vi "24路数据解析例程.vi"() -> ()   [LabVIEW 2018]
panel:
  in  "16进制":bool
  in  "返回数据（字符串）":string
  out "LED IrCompare Result":u8[][](array[numeric])
  out "LED VfCompare Result":u8[][](array[numeric])
  out "LED IrResult":sgl[][](array[numeric]) format="%#_6f"
  out "LED VfResult":sgl[][](array[numeric]) format="%#_6f"
  out "Bls Result":sgl[][](array[numeric]) format="%#_6f"
  out "总判断":u8
  out "PS Compare Result":u8[][](array[numeric])
  out "Balance Compare Result":u8[][](array[numeric])
  out "Z Compare Result":u8[][](array[numeric])
  out "Rs Compare Result":u8[][](array[numeric])
  out "LxQ Compare Result":u8[][](array[numeric])
  out "DCR Compare Result":u8[][](array[numeric])
  out "C Compare Result":u8[][](array[numeric])
  out "Lk Compare Result":u8[][](array[numeric])
  out "Lx Compare Result":u8[][](array[numeric])
  out "Turns Compare Result":u8[][](array[numeric])
  out "Polarity Result1":string[][](array[string])
  out "Polarity Result":u8[][](array[numeric])
  out "Zx Result":sgl[][](array[numeric]) format="%#_6f"
  out "ACR Result":sgl[][](array[numeric]) format="%#_6f"
  out "LxQ Result":sgl[][](array[numeric]) format="%#_6f"
  out "DCR Result":sgl[][](array[numeric]) format="%#_6f"
  out "Cx Result":sgl[][](array[numeric]) format="%#_6f"
  out "Lk Result":sgl[][](array[numeric]) format="%#_6f"
  out "Lx Result":sgl[][](array[numeric]) format="%#_6f"
  out "Turns Result":sgl[][](array[numeric]) format="%#_6f"
  out "Primary Sets":string
  out "head":string
  in  "返回数据（16进制字符）":string
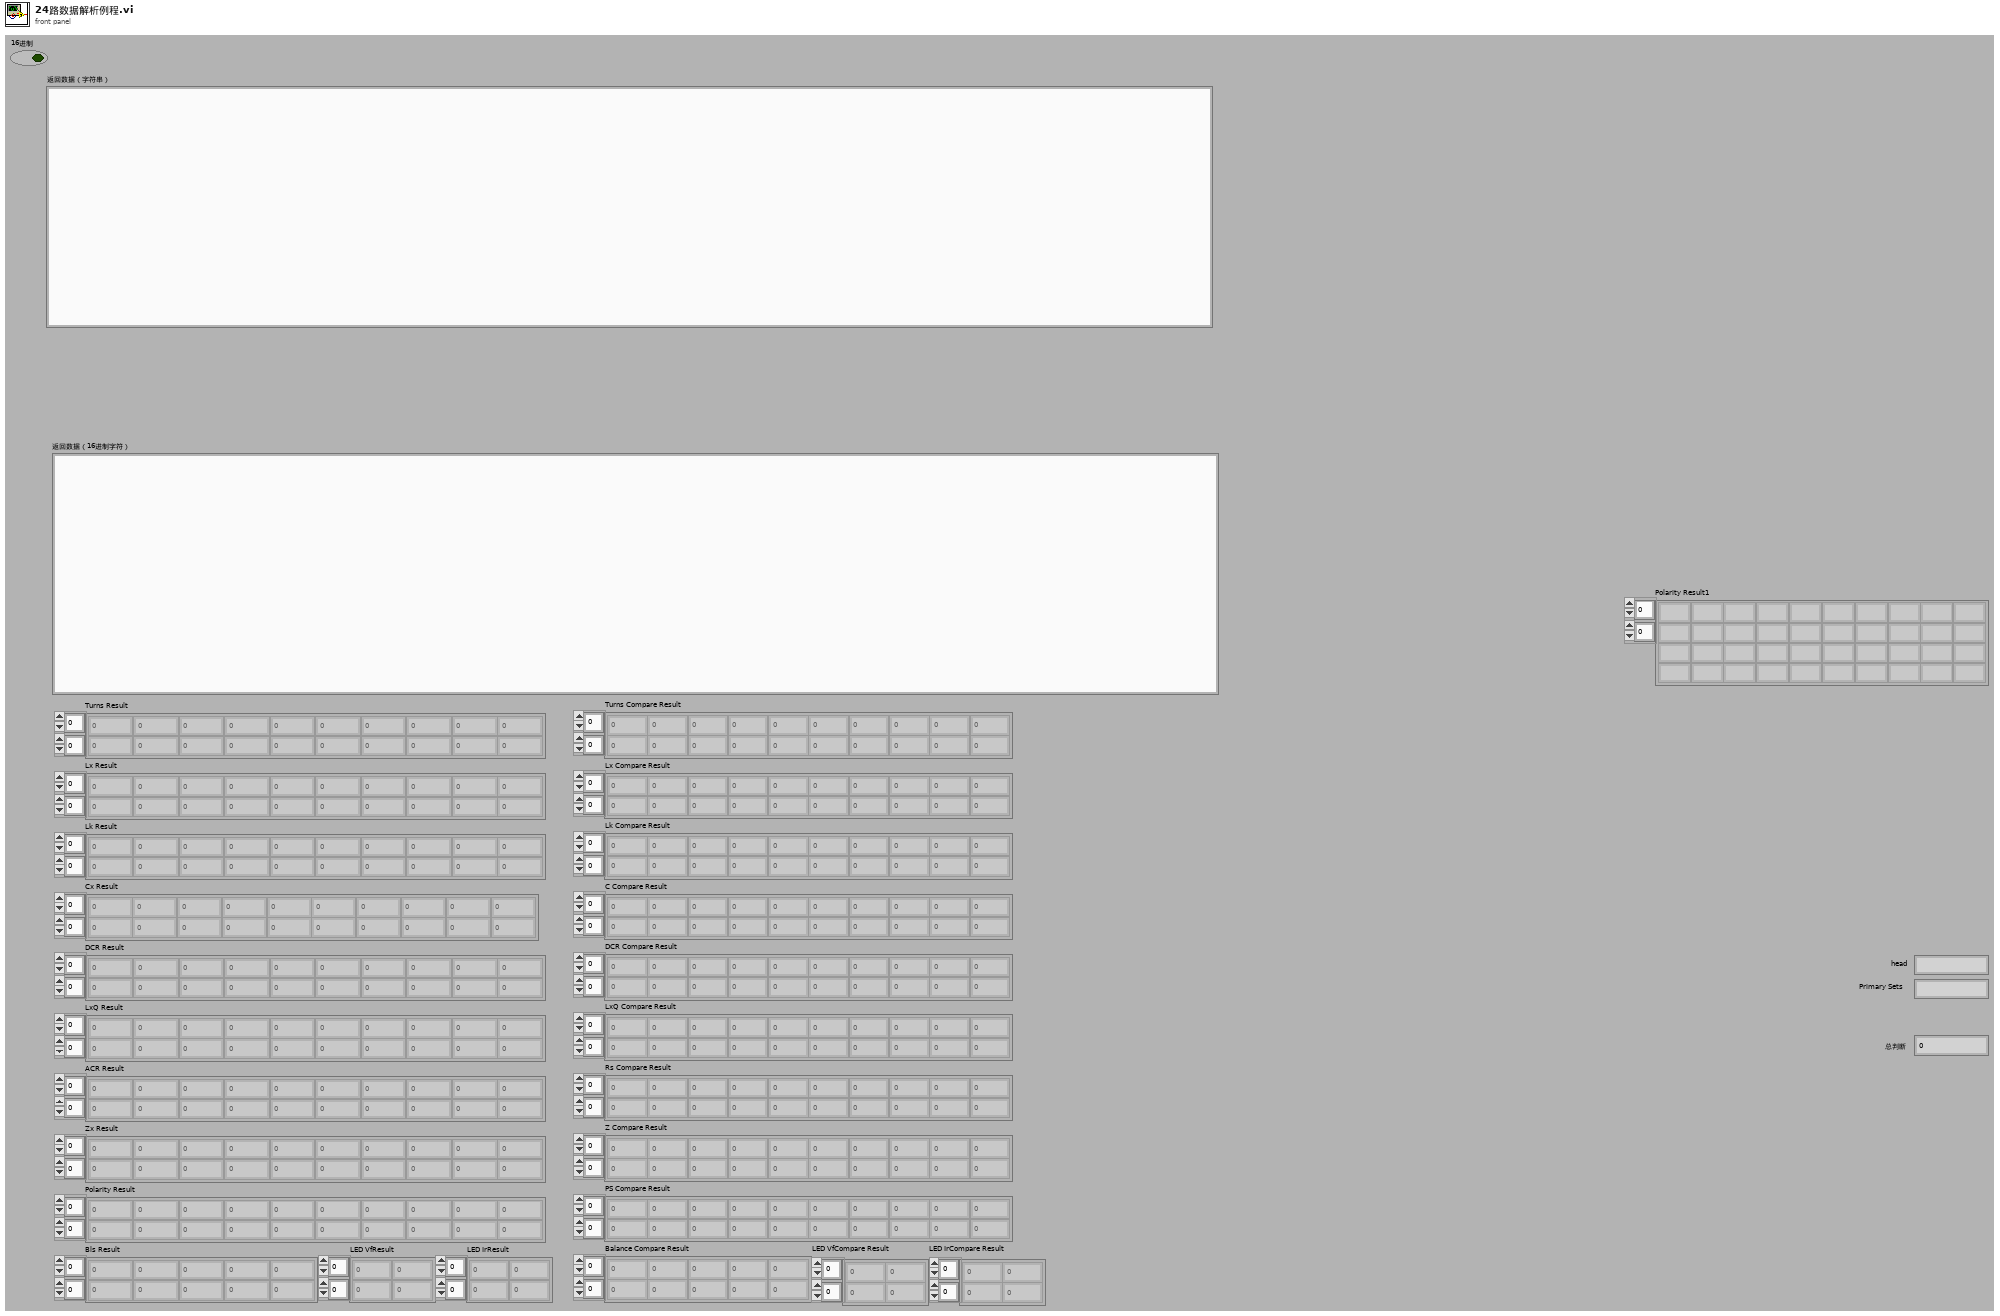
[diagram p1: front panel]
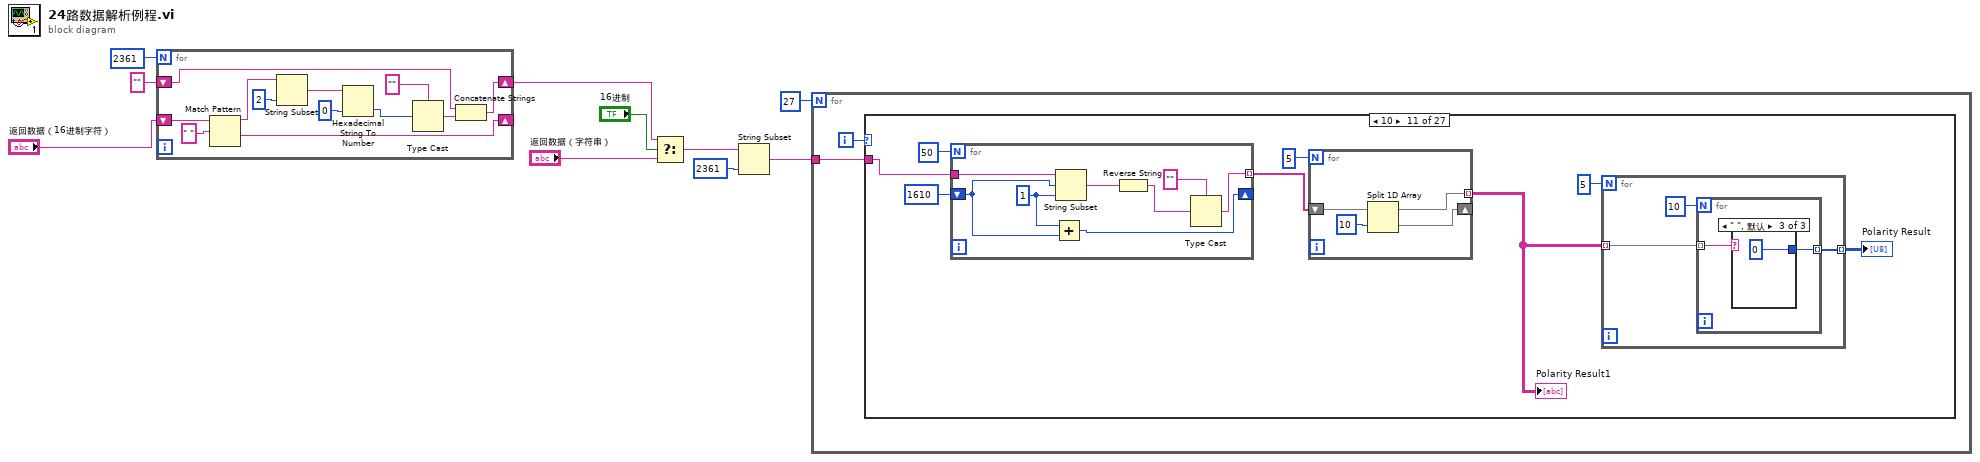
[diagram p0: block diagram]
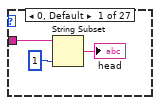
[diagram p2: hidden frame]
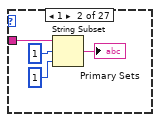
[diagram p3: hidden frame]
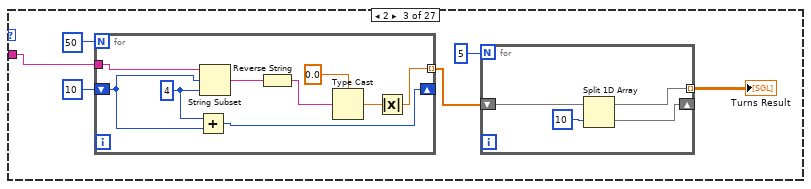
[diagram p4: hidden frame]
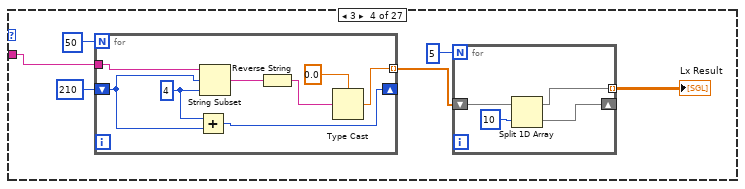
[diagram p5: hidden frame]
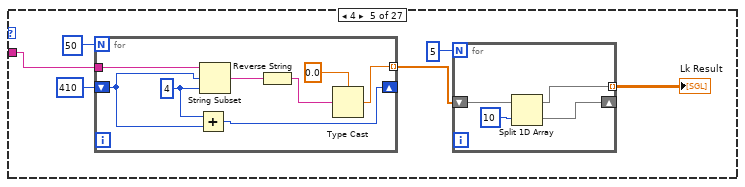
[diagram p6: hidden frame]
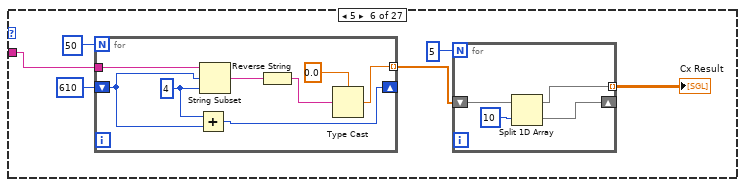
[diagram p7: hidden frame]
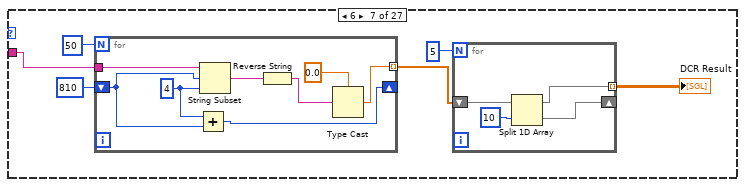
[diagram p8: hidden frame]
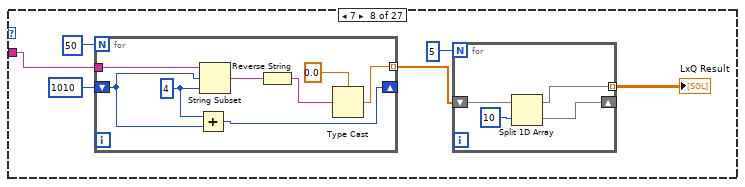
[diagram p9: hidden frame]
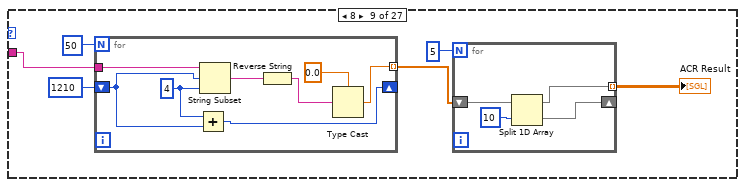
[diagram p10: hidden frame]
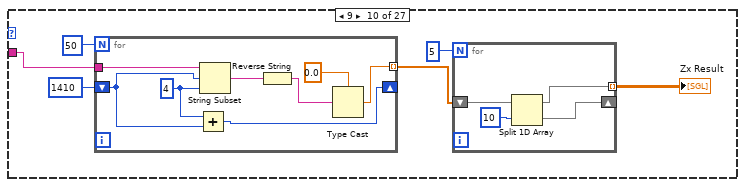
[diagram p11: hidden frame]
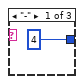
[diagram p12: hidden frame]
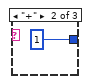
[diagram p13: hidden frame]
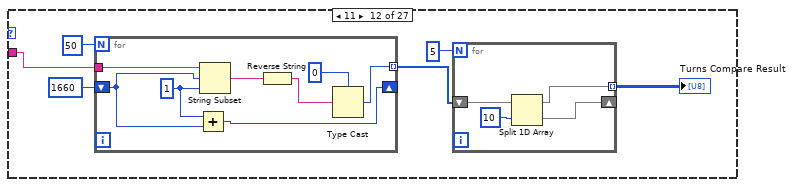
[diagram p14: hidden frame]
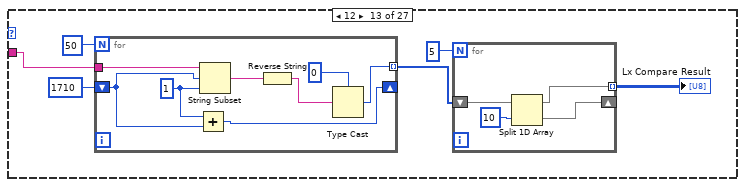
[diagram p15: hidden frame]
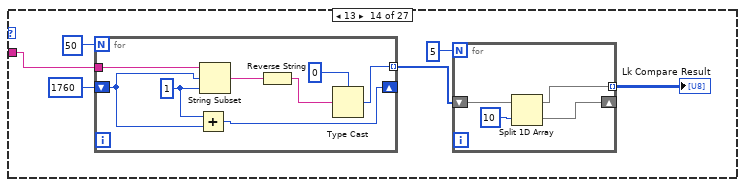
[diagram p16: hidden frame]
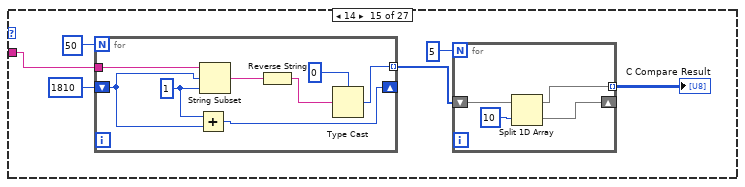
[diagram p17: hidden frame]
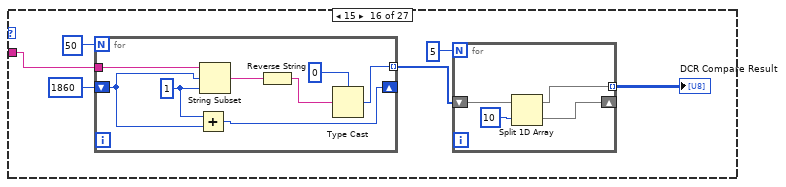
[diagram p18: hidden frame]
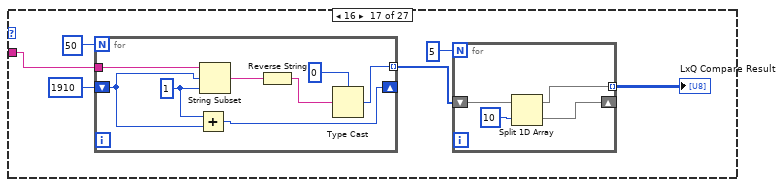
[diagram p19: hidden frame]
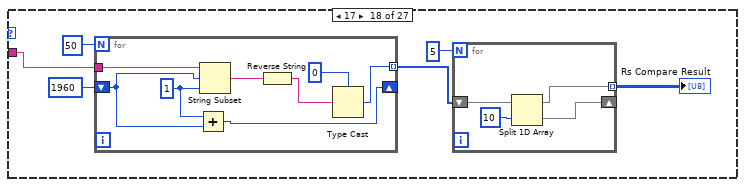
[diagram p20: hidden frame]
diagram:
  n1 = for {
    N: 2361 -> [_]
    shift-right: [w20] -> _
    shift-left: "返回数据（16进制字符）" -> [w22]
    shift-right: [w11] -> w4
    shift-left: "" -> [w13]
    n2 = Match Pattern(string=w22, regular expression=" " ("正则表达式")) -> (before substring=w16:string, after substring=w20:string)  [unwired: 1 in, 2 out]
    n3 = String Subset(string=w16, length (rest)=2 ("长度（剩余）")) -> (substring=w18:string)  [unwired: 1 in]
    n4 = Hexadecimal String To Number(string=w18, default (0uL)=u8 0 ("默认(0 U32)")) -> (number=w14:u8)  [unwired: 1 in, 1 out]
    n5 = Type Cast(type="", x=w14) -> (*(type *) &x=w12:string)
    n6 = Concatenate Strings(w13, w12) -> (w11:string)
  }
  n7 = Select(t=w4, s="16进制", f="返回数据（字符串）") -> (s? t:f=w1:string)
  n8 = String Subset(string=w1, length (rest)=2361 ("长度（剩余）")) -> (substring=w6:string)  [unwired: 1 in]
  n9 = for {
    N: 27 -> [_]
    tunnel: w6 -> [w23]
    i -> [w24]
    n10 = case shown="10" w24 {
      tunnel: w23 -> [w27 w31 w36 w55 w73 w91 w109 w127 w145 w163 w183 w209 w227 w245 w263 w281 w299 w317 w335 w353 w371 w388 w392 w410 w428 w446 w464]
      frame 0, Default {
        n11 = String Subset(string=w27, length (rest)=1 ("长度（剩余）")) -> (substring=→"head":string)  [unwired: 1 in]
      }
      frame 1 {
        n12 = String Subset ("截取字符串")(string=w31, offset (0)=1 ("长度（剩余）"), length (rest)=1 ("长度（剩余）")) -> (substring=→"Primary Sets":string)
      }
      frame 2 {
        n13 = for {
          N: 50 -> [_]
          shift-right: [w46] -> _
          shift-left: 10 ("长度（剩余）") -> [w42]
          tunnel: w36 -> [w41]
          tunnel: [w38] -> w34 mode=indexing
          w43 = 4 ("长度（剩余）")
          n14 = Add(x=w43, y=w42) -> (x+y=w46:i32)
          n15 = String Subset(string=w41, offset (0)=w42, length (rest)=w43) -> (substring=w40:string)
          n16 = Reverse String(1:w40) -> (0:w45:string)
          n17 = Type Cast(type=sgl 0.0 ("长度（剩余）"), x=w45) -> (*(type *) &x=w39:sgl)
          n18 = Absolute Value(x=w39) -> (abs(x)=w38:sgl)
        }
        n19 = for {
          N: 5 -> [_]
          shift-right: [w49] -> _
          shift-left: w34 -> [w47]
          tunnel: [w48] -> w32 mode=indexing
          n20 = Split 1D Array(array=w47, index=10 ("索引")) -> (first subarray=w48:sgl[], second subarray=w49:sgl[])
        }
        "Turns Result" <- w32
      }
      frame 3 {
        n21 = for {
          N: 50 -> [_]
          shift-right: [w64] -> _
          shift-left: 210 ("长度（剩余）") -> [w60]
          tunnel: w55 -> [w59]
          tunnel: [w57] -> w53 mode=indexing
          w61 = 4 ("长度（剩余）")
          n22 = Add(x=w61, y=w60) -> (x+y=w64:i32)
          n23 = String Subset(string=w59, offset (0)=w60, length (rest)=w61) -> (substring=w58:string)
          n24 = Reverse String(1:w58) -> (0:w63:string)
          n25 = Type Cast(type=sgl 0.0 ("长度（剩余）"), x=w63) -> (*(type *) &x=w57:sgl)
        }
        n26 = for {
          N: 5 -> [_]
          shift-right: [w67] -> _
          shift-left: w53 -> [w65]
          tunnel: [w66] -> w51 mode=indexing
          n27 = Split 1D Array(array=w65, index=10 ("索引")) -> (first subarray=w66:sgl[], second subarray=w67:sgl[])
        }
        "Lx Result" <- w51
      }
      frame 4 {
        n28 = for {
          N: 50 -> [_]
          shift-right: [w82] -> _
          shift-left: 410 ("长度（剩余）") -> [w78]
          tunnel: w73 -> [w77]
          tunnel: [w75] -> w71 mode=indexing
          w79 = 4 ("长度（剩余）")
          n29 = Add(x=w79, y=w78) -> (x+y=w82:i32)
          n30 = String Subset(string=w77, offset (0)=w78, length (rest)=w79) -> (substring=w76:string)
          n31 = Reverse String(1:w76) -> (0:w81:string)
          n32 = Type Cast(type=sgl 0.0 ("长度（剩余）"), x=w81) -> (*(type *) &x=w75:sgl)
        }
        n33 = for {
          N: 5 -> [_]
          shift-right: [w85] -> _
          shift-left: w71 -> [w83]
          tunnel: [w84] -> w69 mode=indexing
          n34 = Split 1D Array(array=w83, index=10 ("索引")) -> (first subarray=w84:sgl[], second subarray=w85:sgl[])
        }
        "Lk Result" <- w69
      }
      frame 5 {
        n35 = for {
          N: 50 -> [_]
          shift-right: [w100] -> _
          shift-left: 610 ("长度（剩余）") -> [w96]
          tunnel: w91 -> [w95]
          tunnel: [w93] -> w89 mode=indexing
          w97 = 4 ("长度（剩余）")
          n36 = Add(x=w97, y=w96) -> (x+y=w100:i32)
          n37 = String Subset(string=w95, offset (0)=w96, length (rest)=w97) -> (substring=w94:string)
          n38 = Reverse String(1:w94) -> (0:w99:string)
          n39 = Type Cast(type=sgl 0.0 ("长度（剩余）"), x=w99) -> (*(type *) &x=w93:sgl)
        }
        n40 = for {
          N: 5 -> [_]
          shift-right: [w103] -> _
          shift-left: w89 -> [w101]
          tunnel: [w102] -> w87 mode=indexing
          n41 = Split 1D Array(array=w101, index=10 ("索引")) -> (first subarray=w102:sgl[], second subarray=w103:sgl[])
        }
        "Cx Result" <- w87
      }
      frame 6 {
        n42 = for {
          N: 50 -> [_]
          shift-right: [w118] -> _
          shift-left: 810 ("长度（剩余）") -> [w114]
          tunnel: w109 -> [w113]
          tunnel: [w111] -> w107 mode=indexing
          w115 = 4 ("长度（剩余）")
          n43 = Add(x=w115, y=w114) -> (x+y=w118:i32)
          n44 = String Subset(string=w113, offset (0)=w114, length (rest)=w115) -> (substring=w112:string)
          n45 = Reverse String(1:w112) -> (0:w117:string)
          n46 = Type Cast(type=sgl 0.0 ("长度（剩余）"), x=w117) -> (*(type *) &x=w111:sgl)
        }
        n47 = for {
          N: 5 -> [_]
          shift-right: [w121] -> _
          shift-left: w107 -> [w119]
          tunnel: [w120] -> w105 mode=indexing
          n48 = Split 1D Array(array=w119, index=10 ("索引")) -> (first subarray=w120:sgl[], second subarray=w121:sgl[])
        }
        "DCR Result" <- w105
      }
      frame 7 {
        n49 = for {
          N: 50 -> [_]
          shift-right: [w136] -> _
          shift-left: 1010 ("长度（剩余）") -> [w132]
          tunnel: w127 -> [w131]
          tunnel: [w129] -> w125 mode=indexing
          w133 = 4 ("长度（剩余）")
          n50 = Add(x=w133, y=w132) -> (x+y=w136:i32)
          n51 = String Subset(string=w131, offset (0)=w132, length (rest)=w133) -> (substring=w130:string)
          n52 = Reverse String(1:w130) -> (0:w135:string)
          n53 = Type Cast(type=sgl 0.0 ("长度（剩余）"), x=w135) -> (*(type *) &x=w129:sgl)
        }
        n54 = for {
          N: 5 -> [_]
          shift-right: [w139] -> _
          shift-left: w125 -> [w137]
          tunnel: [w138] -> w123 mode=indexing
          n55 = Split 1D Array(array=w137, index=10 ("索引")) -> (first subarray=w138:sgl[], second subarray=w139:sgl[])
        }
        "LxQ Result" <- w123
      }
      frame 8 {
        n56 = for {
          N: 50 -> [_]
          shift-right: [w154] -> _
          shift-left: 1210 ("长度（剩余）") -> [w150]
          tunnel: w145 -> [w149]
          tunnel: [w147] -> w143 mode=indexing
          w151 = 4 ("长度（剩余）")
          n57 = Add(x=w151, y=w150) -> (x+y=w154:i32)
          n58 = String Subset(string=w149, offset (0)=w150, length (rest)=w151) -> (substring=w148:string)
          n59 = Reverse String(1:w148) -> (0:w153:string)
          n60 = Type Cast(type=sgl 0.0 ("长度（剩余）"), x=w153) -> (*(type *) &x=w147:sgl)
        }
        n61 = for {
          N: 5 -> [_]
          shift-right: [w157] -> _
          shift-left: w143 -> [w155]
          tunnel: [w156] -> w141 mode=indexing
          n62 = Split 1D Array(array=w155, index=10 ("索引")) -> (first subarray=w156:sgl[], second subarray=w157:sgl[])
        }
        "ACR Result" <- w141
      }
      frame 9 {
        n63 = for {
          N: 50 -> [_]
          shift-right: [w172] -> _
          shift-left: 1410 ("长度（剩余）") -> [w168]
          tunnel: w163 -> [w167]
          tunnel: [w165] -> w161 mode=indexing
          w169 = 4 ("长度（剩余）")
          n64 = Add(x=w169, y=w168) -> (x+y=w172:i32)
          n65 = String Subset(string=w167, offset (0)=w168, length (rest)=w169) -> (substring=w166:string)
          n66 = Reverse String(1:w166) -> (0:w171:string)
          n67 = Type Cast(type=sgl 0.0 ("长度（剩余）"), x=w171) -> (*(type *) &x=w165:sgl)
        }
        n68 = for {
          N: 5 -> [_]
          shift-right: [w175] -> _
          shift-left: w161 -> [w173]
          tunnel: [w174] -> w159 mode=indexing
          n69 = Split 1D Array(array=w173, index=10 ("索引")) -> (first subarray=w174:sgl[], second subarray=w175:sgl[])
        }
        "Zx Result" <- w159
      }
      frame 10 {
        n70 = for {
          N: 50 -> [_]
          shift-right: [w200] -> _
          shift-left: 1610 ("长度（剩余）") -> [w197]
          tunnel: w183 -> [w196]
          tunnel: [w194] -> w178 mode=indexing
          w198 = 1 ("长度（剩余）")
          n71 = Add(x=w198, y=w197) -> (x+y=w200:i32)
          n72 = String Subset(string=w196, offset (0)=w197, length (rest)=w198) -> (substring=w195:string)
          n73 = Reverse String(1:w195) -> (0:w199:string)
          n74 = Type Cast(type="", x=w199) -> (*(type *) &x=w194:string)
        }
        n75 = for {
          N: 5 -> [_]
          shift-right: [w203] -> _
          shift-left: w178 -> [w201]
          tunnel: [w202] -> w177 mode=indexing
          n76 = Split 1D Array(array=w201, index=10 ("索引")) -> (first subarray=w202:string[], second subarray=w203:string[])
        }
        "Polarity Result1" <- w177
        n77 = for {
          N: 5 -> [_]
          tunnel: w177 -> [w186] mode=indexing
          tunnel: [w185] -> w179 mode=indexing
          n78 = for {
            N: 10 -> [_]
            tunnel: w186 -> [w189] mode=indexing
            tunnel: [w188] -> w185 mode=indexing
            n79 = case shown="\" \", 默认" w189 {
              tunnel: [u8 4 u8 1 u8 0] -> w188
              frame "-" {
              }
              frame "+" {
              }
              frame " ", Default {
              }
            }
          }
        }
        "Polarity Result" <- w179
      }
      frame 11 {
        n80 = for {
          N: 50 -> [_]
          shift-right: [w218] -> _
          shift-left: 1660 ("长度（剩余）") -> [w214]
          tunnel: w209 -> [w213]
          tunnel: [w211] -> w207 mode=indexing
          w215 = 1 ("长度（剩余）")
          n81 = Add(x=w215, y=w214) -> (x+y=w218:i32)
          n82 = String Subset ("截取字符串")(string=w213, offset (0)=w214, length (rest)=w215) -> (substring=w212:string)
          n83 = Reverse String(1:w212) -> (0:w217:string)
          n84 = Type Cast(type=u8 0 ("长度（剩余）"), x=w217) -> (*(type *) &x=w211:u8)
        }
        n85 = for {
          N: 5 -> [_]
          shift-right: [w221] -> _
          shift-left: w207 -> [w219]
          tunnel: [w220] -> w205 mode=indexing
          n86 = Split 1D Array(array=w219, index=10 ("索引")) -> (first subarray=w220:u8[], second subarray=w221:u8[])
        }
        "Turns Compare Result" <- w205
      }
      frame 12 {
        n87 = for {
          N: 50 -> [_]
          shift-right: [w236] -> _
          shift-left: 1710 ("长度（剩余）") -> [w232]
          tunnel: w227 -> [w231]
          tunnel: [w229] -> w225 mode=indexing
          w233 = 1 ("长度（剩余）")
          n88 = Add(x=w233, y=w232) -> (x+y=w236:i32)
          n89 = String Subset(string=w231, offset (0)=w232, length (rest)=w233) -> (substring=w230:string)
          n90 = Reverse String(1:w230) -> (0:w235:string)
          n91 = Type Cast(type=u8 0 ("长度（剩余）"), x=w235) -> (*(type *) &x=w229:u8)
        }
        n92 = for {
          N: 5 -> [_]
          shift-right: [w239] -> _
          shift-left: w225 -> [w237]
          tunnel: [w238] -> w223 mode=indexing
          n93 = Split 1D Array(array=w237, index=10 ("索引")) -> (first subarray=w238:u8[], second subarray=w239:u8[])
        }
        "Lx Compare Result" <- w223
      }
      frame 13 {
        n94 = for {
          N: 50 -> [_]
          shift-right: [w254] -> _
          shift-left: 1760 ("长度（剩余）") -> [w250]
          tunnel: w245 -> [w249]
          tunnel: [w247] -> w243 mode=indexing
          w251 = 1 ("长度（剩余）")
          n95 = Add(x=w251, y=w250) -> (x+y=w254:i32)
          n96 = String Subset(string=w249, offset (0)=w250, length (rest)=w251) -> (substring=w248:string)
          n97 = Reverse String(1:w248) -> (0:w253:string)
          n98 = Type Cast(type=u8 0 ("长度（剩余）"), x=w253) -> (*(type *) &x=w247:u8)
        }
        n99 = for {
          N: 5 -> [_]
          shift-right: [w257] -> _
          shift-left: w243 -> [w255]
          tunnel: [w256] -> w241 mode=indexing
          n100 = Split 1D Array(array=w255, index=10 ("索引")) -> (first subarray=w256:u8[], second subarray=w257:u8[])
        }
        "Lk Compare Result" <- w241
      }
      frame 14 {
        n101 = for {
          N: 50 -> [_]
          shift-right: [w272] -> _
          shift-left: 1810 ("长度（剩余）") -> [w268]
          tunnel: w263 -> [w267]
          tunnel: [w265] -> w261 mode=indexing
          w269 = 1 ("长度（剩余）")
          n102 = Add(x=w269, y=w268) -> (x+y=w272:i32)
          n103 = String Subset(string=w267, offset (0)=w268, length (rest)=w269) -> (substring=w266:string)
          n104 = Reverse String(1:w266) -> (0:w271:string)
          n105 = Type Cast(type=u8 0 ("长度（剩余）"), x=w271) -> (*(type *) &x=w265:u8)
        }
        n106 = for {
          N: 5 -> [_]
          shift-right: [w275] -> _
          shift-left: w261 -> [w273]
          tunnel: [w274] -> w259 mode=indexing
          n107 = Split 1D Array(array=w273, index=10 ("索引")) -> (first subarray=w274:u8[], second subarray=w275:u8[])
        }
        "C Compare Result" <- w259
      }
      frame 15 {
        n108 = for {
          N: 50 -> [_]
          shift-right: [w290] -> _
          shift-left: 1860 ("长度（剩余）") -> [w286]
          tunnel: w281 -> [w285]
          tunnel: [w283] -> w279 mode=indexing
          w287 = 1 ("长度（剩余）")
          n109 = Add(x=w287, y=w286) -> (x+y=w290:i32)
          n110 = String Subset(string=w285, offset (0)=w286, length (rest)=w287) -> (substring=w284:string)
          n111 = Reverse String(1:w284) -> (0:w289:string)
          n112 = Type Cast(type=u8 0 ("长度（剩余）"), x=w289) -> (*(type *) &x=w283:u8)
        }
        n113 = for {
          N: 5 -> [_]
          shift-right: [w293] -> _
          shift-left: w279 -> [w291]
          tunnel: [w292] -> w277 mode=indexing
          n114 = Split 1D Array(array=w291, index=10 ("索引")) -> (first subarray=w292:u8[], second subarray=w293:u8[])
        }
        "DCR Compare Result" <- w277
      }
      frame 16 {
        n115 = for {
          N: 50 -> [_]
          shift-right: [w308] -> _
          shift-left: 1910 ("长度（剩余）") -> [w304]
          tunnel: w299 -> [w303]
          tunnel: [w301] -> w297 mode=indexing
          w305 = 1 ("长度（剩余）")
          n116 = Add(x=w305, y=w304) -> (x+y=w308:i32)
          n117 = String Subset(string=w303, offset (0)=w304, length (rest)=w305) -> (substring=w302:string)
          n118 = Reverse String(1:w302) -> (0:w307:string)
          n119 = Type Cast(type=u8 0 ("长度（剩余）"), x=w307) -> (*(type *) &x=w301:u8)
        }
        n120 = for {
          N: 5 -> [_]
          shift-right: [w311] -> _
          shift-left: w297 -> [w309]
          tunnel: [w310] -> w295 mode=indexing
          n121 = Split 1D Array(array=w309, index=10 ("索引")) -> (first subarray=w310:u8[], second subarray=w311:u8[])
        }
        "LxQ Compare Result" <- w295
      }
      frame 17 {
        n122 = for {
          N: 50 -> [_]
          shift-right: [w326] -> _
          shift-left: 1960 ("长度（剩余）") -> [w320]
          tunnel: w317 -> [w321]
          tunnel: [w322] -> w315 mode=indexing
          w319 = 1 ("长度（剩余）")
          n123 = Add(x=w319, y=w320) -> (x+y=w326:i32)
          n124 = String Subset(string=w321, offset (0)=w320, length (rest)=w319) -> (substring=w323:string)
          n125 = Reverse String(1:w323) -> (0:w325:string)
          n126 = Type Cast(type=u8 0 ("长度（剩余）"), x=w325) -> (*(type *) &x=w322:u8)
        }
        n127 = for {
          N: 5 -> [_]
          shift-right: [w329] -> _
          shift-left: w315 -> [w327]
          tunnel: [w328] -> w313 mode=indexing
          n128 = Split 1D Array(array=w327, index=10 ("索引")) -> (first subarray=w328:u8[], second subarray=w329:u8[])
        }
        "Rs Compare Result" <- w313
      }
      frame 18 {
        n129 = for {
          N: 50 -> [_]
          shift-right: [w344] -> _
          shift-left: 2010 ("长度（剩余）") -> [w338]
          tunnel: w335 -> [w339]
          tunnel: [w340] -> w333 mode=indexing
          w337 = 1 ("长度（剩余）")
          n130 = Add(x=w337, y=w338) -> (x+y=w344:i32)
          n131 = String Subset(string=w339, offset (0)=w338, length (rest)=w337) -> (substring=w341:string)
          n132 = Reverse String(1:w341) -> (0:w343:string)
          n133 = Type Cast(type=u8 0 ("长度（剩余）"), x=w343) -> (*(type *) &x=w340:u8)
        }
        n134 = for {
          N: 5 -> [_]
          shift-right: [w347] -> _
          shift-left: w333 -> [w345]
          tunnel: [w346] -> w331 mode=indexing
          n135 = Split 1D Array(array=w345, index=10 ("索引")) -> (first subarray=w346:u8[], second subarray=w347:u8[])
        }
        "Z Compare Result" <- w331
      }
      frame 19 {
        n136 = for {
          N: 50 -> [_]
          shift-right: [w362] -> _
          shift-left: 2060 ("长度（剩余）") -> [w357]
          tunnel: w353 -> [w358]
          tunnel: [w359] -> w351 mode=indexing
          w356 = 1 ("长度（剩余）")
          n137 = Add(x=w356, y=w357) -> (x+y=w362:i32)
          n138 = String Subset(string=w358, offset (0)=w357, length (rest)=w356) -> (substring=w360:string)
          n139 = Reverse String(1:w360) -> (0:w361:string)
          n140 = Type Cast(type=u8 0 ("长度（剩余）"), x=w361) -> (*(type *) &x=w359:u8)
        }
        n141 = for {
          N: 5 -> [_]
          shift-right: [w365] -> _
          shift-left: w351 -> [w363]
          tunnel: [w364] -> w349 mode=indexing
          n142 = Split 1D Array(array=w363, index=10 ("索引")) -> (first subarray=w364:u8[], second subarray=w365:u8[])
        }
        "Balance Compare Result" <- w349
      }
      frame 20 {
        n143 = for {
          N: 50 -> [_]
          shift-right: [w380] -> _
          shift-left: 2110 ("长度（剩余）") -> [w375]
          tunnel: w371 -> [w376]
          tunnel: [w377] -> w369 mode=indexing
          w374 = 1 ("长度（剩余）")
          n144 = Add(x=w374, y=w375) -> (x+y=w380:i32)
          n145 = String Subset(string=w376, offset (0)=w375, length (rest)=w374) -> (substring=w378:string)
          n146 = Reverse String(1:w378) -> (0:w379:string)
          n147 = Type Cast(type=u8 0 ("长度（剩余）"), x=w379) -> (*(type *) &x=w377:u8)
        }
        n148 = for {
          N: 5 -> [_]
          shift-right: [w383] -> _
          shift-left: w369 -> [w381]
          tunnel: [w382] -> w367 mode=indexing
          n149 = Split 1D Array(array=w381, index=10 ("索引")) -> (first subarray=w382:u8[], second subarray=w383:u8[])
        }
        "PS Compare Result" <- w367
      }
      frame 21 {
        n150 = String Subset(string=w388, offset (0)=2160 ("长度（剩余）"), length (rest)=1 ("长度（剩余）")) -> (substring=w391:string)
        n151 = Reverse String(1:w391) -> (0:w389:string)
        n152 = Type Cast(type=u8 0 ("长度（剩余）"), x=w389) -> (*(type *) &x=→"总判断":u8)
      }
      frame 22 {
        n153 = for {
          N: 25 -> [_]
          shift-right: [w405] -> _
          shift-left: 2161 ("长度（剩余）") -> [w401]
          tunnel: w392 -> [w400]
          tunnel: [w398] -> w395 mode=indexing
          w402 = 4 ("长度（剩余）")
          n154 = Add(x=w402, y=w401) -> (x+y=w405:i32)
          n155 = String Subset(string=w400, offset (0)=w401, length (rest)=w402) -> (substring=w399:string)
          n156 = Reverse String(1:w399) -> (0:w404:string)
          n157 = Type Cast(type=sgl 0.0 ("长度（剩余）"), x=w404) -> (*(type *) &x=w398:sgl)
        }
        n158 = for {
          N: 5 -> [_]
          shift-right: [w408] -> _
          shift-left: w395 -> [w406]
          tunnel: [w407] -> w393 mode=indexing
          n159 = Split 1D Array(array=w406, index=5 ("索引")) -> (first subarray=w407:sgl[], second subarray=w408:sgl[])
        }
        "Bls Result" <- w393
      }
      frame 23 {
        n160 = for {
          N: 10 -> [_]
          shift-right: [w423] -> _
          shift-left: 2261 ("长度（剩余）") -> [w419]
          tunnel: w410 -> [w418]
          tunnel: [w416] -> w412 mode=indexing
          w420 = 4 ("长度（剩余）")
          n161 = Add(x=w420, y=w419) -> (x+y=w423:i32)
          n162 = String Subset(string=w418, offset (0)=w419, length (rest)=w420) -> (substring=w417:string)
          n163 = Reverse String(1:w417) -> (0:w422:string)
          n164 = Type Cast(type=sgl 0.0 ("长度（剩余）"), x=w422) -> (*(type *) &x=w416:sgl)
        }
        n165 = for {
          N: 5 -> [_]
          shift-right: [w426] -> _
          shift-left: w412 -> [w424]
          tunnel: [w425] -> w415 mode=indexing
          n166 = Split 1D Array(array=w424, index=2 ("索引")) -> (first subarray=w425:sgl[], second subarray=w426:sgl[])
        }
        "LED VfResult" <- w415
      }
      frame 24 {
        n167 = for {
          N: 10 -> [_]
          shift-right: [w441] -> _
          shift-left: 2301 ("长度（剩余）") -> [w437]
          tunnel: w428 -> [w436]
          tunnel: [w434] -> w430 mode=indexing
          w438 = 4 ("长度（剩余）")
          n168 = Add(x=w438, y=w437) -> (x+y=w441:i32)
          n169 = String Subset(string=w436, offset (0)=w437, length (rest)=w438) -> (substring=w435:string)
          n170 = Reverse String(1:w435) -> (0:w440:string)
          n171 = Type Cast(type=sgl 0.0 ("长度（剩余）"), x=w440) -> (*(type *) &x=w434:sgl)
        }
        n172 = for {
          N: 5 -> [_]
          shift-right: [w444] -> _
          shift-left: w430 -> [w442]
          tunnel: [w443] -> w433 mode=indexing
          n173 = Split 1D Array(array=w442, index=2 ("索引")) -> (first subarray=w443:sgl[], second subarray=w444:sgl[])
        }
        "LED IrResult" <- w433
      }
      frame 25 {
        n174 = for {
          N: 10 -> [_]
          shift-right: [w459] -> _
          shift-left: 2341 ("长度（剩余）") -> [w454]
          tunnel: w446 -> [w455]
          tunnel: [w456] -> w448 mode=indexing
          w453 = 1 ("长度（剩余）")
          n175 = Add(x=w453, y=w454) -> (x+y=w459:i32)
          n176 = String Subset(string=w455, offset (0)=w454, length (rest)=w453) -> (substring=w457:string)
          n177 = Reverse String(1:w457) -> (0:w458:string)
          n178 = Type Cast(type=u8 0 ("长度（剩余）"), x=w458) -> (*(type *) &x=w456:u8)
        }
        n179 = for {
          N: 5 -> [_]
          shift-right: [w462] -> _
          shift-left: w448 -> [w460]
          tunnel: [w461] -> w451 mode=indexing
          n180 = Split 1D Array(array=w460, index=2 ("索引")) -> (first subarray=w461:u8[], second subarray=w462:u8[])
        }
        "LED VfCompare Result" <- w451
      }
      frame 26 {
        n181 = for {
          N: 10 -> [_]
          shift-right: [w477] -> _
          shift-left: 2351 ("长度（剩余）") -> [w472]
          tunnel: w464 -> [w473]
          tunnel: [w474] -> w466 mode=indexing
          w471 = 1 ("长度（剩余）")
          n182 = Add(x=w471, y=w472) -> (x+y=w477:i32)
          n183 = String Subset(string=w473, offset (0)=w472, length (rest)=w471) -> (substring=w475:string)
          n184 = Reverse String(1:w475) -> (0:w476:string)
          n185 = Type Cast(type=u8 0 ("长度（剩余）"), x=w476) -> (*(type *) &x=w474:u8)
        }
        n186 = for {
          N: 5 -> [_]
          shift-right: [w480] -> _
          shift-left: w466 -> [w478]
          tunnel: [w479] -> w469 mode=indexing
          n187 = Split 1D Array(array=w478, index=2 ("索引")) -> (first subarray=w479:u8[], second subarray=w480:u8[])
        }
        "LED IrCompare Result" <- w469
      }
    }
  }
